vi "Get String.vi"(6 "Don't Create New Tag":bool, 7 "Tag Group":string="Default", 8 "error in (no error)":errorcluster, 10 "Tag":string, 11 "Blackboard in":refnum<class "Blackboard.lvclass">) -> (0 "error out":errorcluster, 1 "New Tag?":bool, 2 "Value":refnum<class "Abs_String.lvclass">, 3 "Blackboard out":refnum<class "Blackboard.lvclass">)   [LabVIEW 2021, in "Blackboard.lvclass"]
uses:
  Blackboard.lvclass
  <vilib>/TSA/Abstract Data Classes/Abs_Types/String/Abs_String.lvclass
  <vilib>/Utility/Data Type/Type Definitions/Data Type.ctl
  Blackboard.lvclass/Blackboard.ctl
  <vilib>/TSA/Omni-Bus/Local Bus/Support/STR/Local Bus_String.lvclass
  C:/Program Files (x86)/National Instruments/LabVIEW 2021/vi.lib/TSA/Abstract Data Classes/Abs_Types/Value/Abs_Value.lvclass
  <vilib>/TSA/Omni-Bus/Local Bus/Support/Initialise DVR's.vi
  <vilib>/TSA/Abstract Data Classes/Abs_Types/Value/Abs_Value.lvclass
  <vilib>/TSA/Abstract Data Classes/Abs_Types/Type/Abs_Type.lvclass
  <vilib>/TSA/Omni-Bus/Local Bus/Support/DBL/Local Bus_DBL.lvclass
  <vilib>/TSA/Omni-Bus/Local Bus/Support/SGL/Local Bus_SGL.lvclass
  <vilib>/TSA/Omni-Bus/Local Bus/Support/EXT/Local Bus_EXT.lvclass
  <vilib>/TSA/Omni-Bus/Local Bus/Support/Bool/Local Bus_Boolean.lvclass
  <vilib>/TSA/Omni-Bus/Local Bus/Support/Variant/Local Bus_Variant.lvclass
  <vilib>/TSA/Omni-Bus/Local Bus/Support/WFM/Local Bus_Waveform.lvclass
  <vilib>/TSA/Omni-Bus/Local Bus/Support/Time/Local Bus_Time.lvclass
  <vilib>/TSA/Omni-Bus/Local Bus/Support/U8/Local Bus_U8.lvclass
  <vilib>/TSA/Omni-Bus/Local Bus/Support/U16/Local Bus_U16.lvclass
  <vilib>/TSA/Omni-Bus/Local Bus/Support/U32/Local Bus_U32.lvclass
  <vilib>/TSA/Omni-Bus/Local Bus/Support/U64/Local Bus_U64.lvclass
  <vilib>/TSA/Omni-Bus/Local Bus/Support/I8/Local Bus_I8.lvclass
  <vilib>/TSA/Omni-Bus/Local Bus/Support/I16/Local Bus_I16.lvclass
  <vilib>/TSA/Omni-Bus/Local Bus/Support/I32/Local Bus_I32.lvclass
  <vilib>/TSA/Omni-Bus/Local Bus/Support/I64/Local Bus_I64.lvclass
  <vilib>/TSA/Omni-Bus/Local Bus/Support/CSGL/Local Bus_CSGL.lvclass
  <vilib>/TSA/Omni-Bus/Local Bus/Support/CDBL/Local Bus_CDBL.lvclass
  <vilib>/TSA/Omni-Bus/Local Bus/Support/CEXT/Local Bus_CEXT.lvclass
  <vilib>/Utility/Data Type/NI_Data Type.lvlib
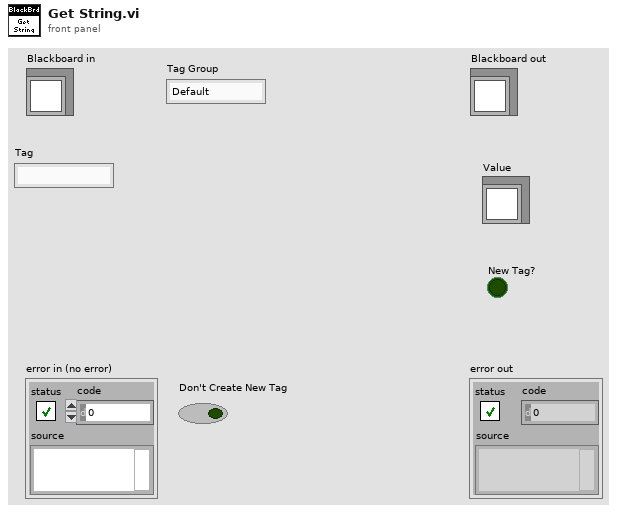
[diagram p1: front panel]
types:
  T1 = typedef "NI_Data Type.lvlib/Data Type.ctl" = enum8{"Invalid Type", "Void", "I8", "I16", "I32", "I64", "U8", "U16", "U32", "U64", "Single Float", "Double Float", "Extended Float", "Single Complex", "Double Complex", "Extended Complex", "Enum U8", "Enum U16", "Enum U32", "Enum U64", "Single Float With Unit", "Double Float With Unit", "Extended Float With Unit", "Single Complex with Unit", "Double Complex with Unit", "Extended Complex with Unit", "Boolean", "String", "Path", "Picture", "Tag", "Array", "Cluster", "Variant", "LV Variant", "Waveform", "Timestamp", "Digital Waveform", "Digital Data", "ExpressData", "Refnum", "External Data", "VI", "Poly VI", "LabVIEW Class Instance", "Fixed Point", "Set Collection", "Map Collection"}
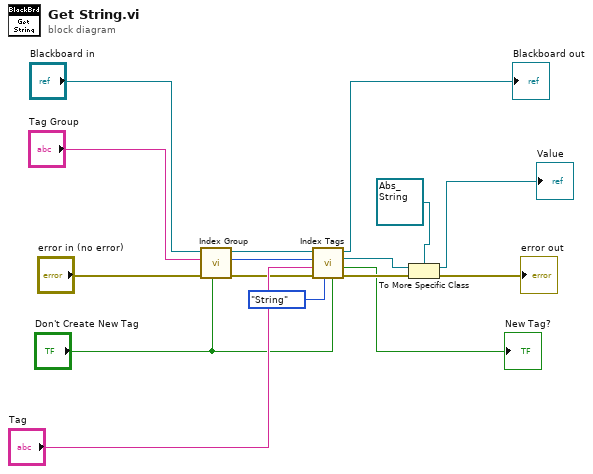
[diagram p0: block diagram]
diagram:
  n1 = call "Index Group.vi"("Don't Create"="Don't Create New Tag", "error in (no error)"="error in (no error)", "Group"="Tag Group", "bt_Blackboard in"="Blackboard in") -> ("error out"=w9:errorcluster, "Index"=w8:i32, "bt_Blackboard out"=w10:refnum<class "Blackboard.lvclass">)  [unwired: 5 in]
  n2 = call "Index Tags.vi"("Don't Create"="Don't Create New Tag", "Tag Type"=Data_Type."String", "error in (no error)"=w9, "Tag"="Tag", "Group Index"=w8, "bt_Blackboard in"=w10) -> ("error out"=w6:errorcluster, "New Tag?"=→"New Tag?":bool, "Value"=w5:refnum<class "Abs_Value.lvclass">, "bt_Blackboard out"=→"Blackboard out":refnum<class "Blackboard.lvclass">)  [unwired: 2 in]
  n3 = To More Specific Class(target class=refnum<class "Abs_String.lvclass"> refnum ("Abs_String.lvclass"), reference=w5, error in=w6) -> (specific class reference=→"Value":refnum<class "Abs_String.lvclass">, error out=→"error out":errorcluster)
